vi "split_and_dequeue_string.vi"(8 "error in (no error)":errorcluster, 11 "queue in":refnum<queue>) -> (0 "error out":errorcluster, 1 "Message Data":variant, 2 "Message":string, 3 "queue out":refnum<queue>)   [LabVIEW 2024]
uses:
  Message Cluster.ctl
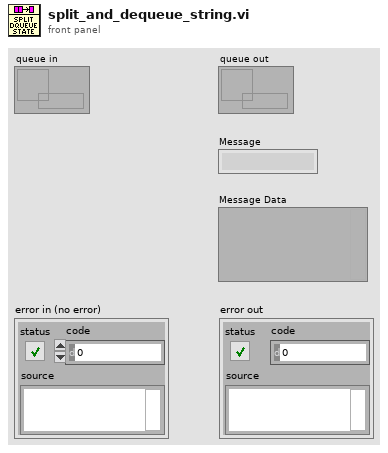
[diagram p1: front panel]
types:
  T1 = typedef "Message Cluster.ctl" = cluster{"Message":string, "Message Data":variant}
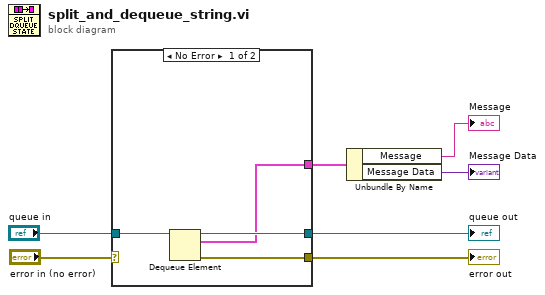
[diagram p0: block diagram]
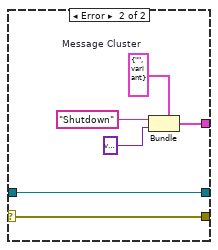
[diagram p2: hidden frame]
diagram:
  n1 = case shown="No Error" "error in (no error)" {
    selector: "error in (no error)" -> [_ w17]
    tunnel: [w11 w17] -> w7
    tunnel: "queue in" -> [w10 w16]
    tunnel: [w9 w16] -> w4
    tunnel: [w8 w13] -> w3
    frame No Error {
      n2 = Dequeue Element(queue=w10) -> (queue out=w9:refnum<queue>, element=w8:T1, error out=w11:errorcluster)  [unwired: 2 in, 1 out]
    }
    frame Error {
      w12 = T1 {"Message"="", "Message Data"=variant}  # Message Cluster
      n3 = Bundle(cluster=w12, "Message"="Shutdown", "Message Data"=variant) -> (w13:T1)
    }
  }
  "error out" <- w7
  "queue out" <- w4
  n4 = Unbundle By Name(w3) -> ("Message"=→"Message":string, "Message Data"=→"Message Data":variant)
